vi "globalSetUp.vi"(8 "error in":errorcluster, 11 "Deployment in":refnum<class "Deployment.lvclass">) -> (0 "error out":errorcluster, 3 "Deployment out":refnum<class "Deployment.lvclass">)   [LabVIEW 2020, in "Deployment.lvclass"]
uses:
  Deployment.lvclass
  Deployment.lvclass/Deployment.ctl
  niveristand-custom-device-testing-tools/VeriStandTestUtilities/VeriStandTestUtilities.lvlib
  Scripting/Ballard MIL-STD-1553 Scripting.lvlib
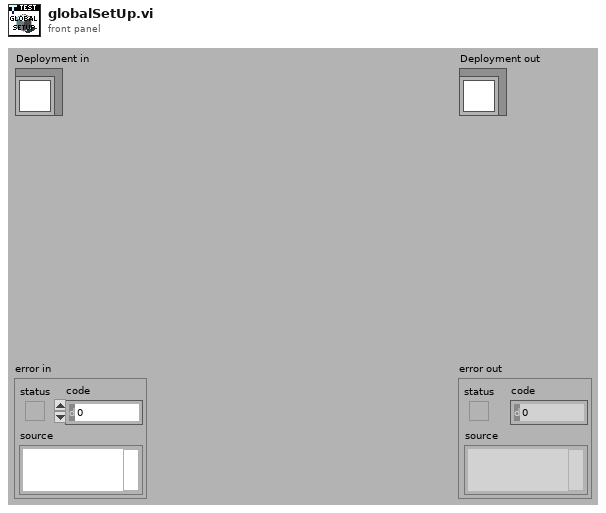
[diagram p1: front panel]
types:
  T1 = typedef "Custom Device API.lvlib/Custom Device Item Ref.ctl" = u64
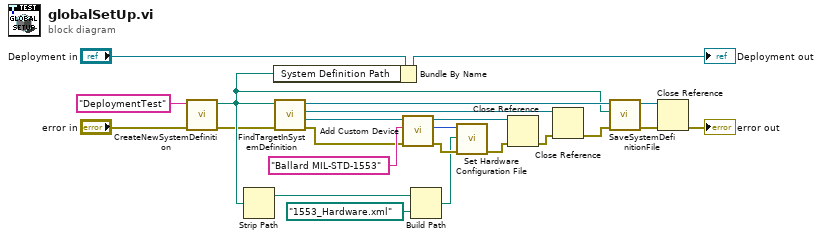
[diagram p0: block diagram]
diagram:
  n1 = call "CreateNewSystemDefinition.vi"("error in"="error in", "System Definition Name"="DeploymentTest") -> ("error out"=w1:errorcluster, "System Definition Path"=w3:path)  [unwired: 8 in]
  n2 = Strip Path(path=w3) -> (stripped path=w8:path)  [unwired: 1 out]
  n3 = Bundle By Name(cluster="Deployment in", "System Definition Path"=w3) -> (→"Deployment out":refnum<class "Deployment.lvclass">)
  n4 = call "FindTargetInSystemDefinition.vi"("error in"=w1, "system definition path"=w3) -> ("error out"=w14:errorcluster, "Target"=w20:refnum<k24>, "Root"=w19:refnum<k24>, "System Definition"=w21:refnum<k24>)  [unwired: 6 in]
  n5 = call "Add Custom Device.vi"("error in"=w14, "name"="Ballard MIL-STD-1553", "target in"=w20) -> ("error out"=w12:errorcluster, "Ballard MIL-STD-1553 custom device"=w13:T1, "target out"=w17:refnum<k24>)  [unwired: 6 in]
  n6 = Build Path(base path=w8, name or relative path=path "1553_Hardware.xml") -> (appended path=w9:path)
  n7 = call "Set Hardware Configuration File.vi"("error in"=w12, "hardware configuration file path"=w9, "Ballard MIL-STD 1553 custom device in"=w13) -> ("error out"=w11:errorcluster)  [unwired: 7 in, 1 out]
  n8 = Close Reference(reference=w17, error in (no error)=w11) -> (error out=w16:errorcluster)
  n9 = Close Reference(reference=w19, error in (no error)=w16) -> (error out=w18:errorcluster)
  n10 = call "SaveSystemDefinitionFile.vi"("error in (no error)"=w18, "System Definition File in"=w3, "System Definition Reference in"=w21) -> ("error out"=w7:errorcluster, "System Definition Reference out"=w5:refnum<k24>)  [unwired: 7 in]
  n11 = Close Reference(reference=w5, error in (no error)=w7) -> (error out=→"error out":errorcluster)
